vi "niRFUtil RFHS Channelizer ClearBuffer CSG.vi"(0 "Buffer":csg[](array[numeric]), 11 "error in (no error)":errorcluster) -> (15 "error out":errorcluster)   [LabVIEW 2015, in "niRFUtil.lvlib"]
uses:
  niRFUtil.lvlib
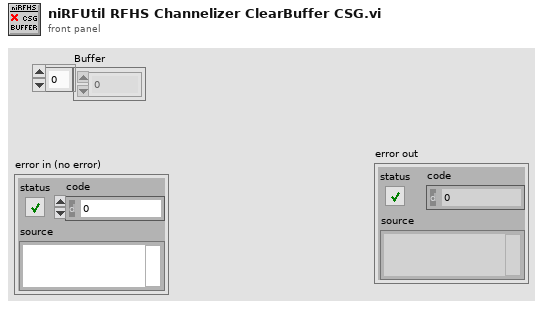
[diagram p1: front panel]
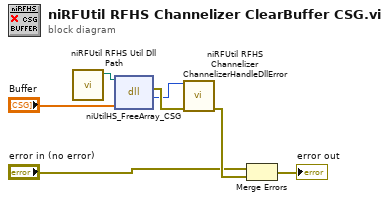
[diagram p0: block diagram]
diagram:
  n1 = call "niRFUtil RFHS Util Dll Path.vi"() -> ("Path"=w6:path)  [unwired: 7 in, 4 out]
  n2 = dll-call lib="?" fn="niUtilHS_FreeArray_CSG"(path in=w6, "buf"="Buffer") -> (error out=w5:errorcluster, "return type"=w4:i32)  [unwired: 3 in, 1 out]
  n3 = call "niRFUtil RFHS Channelizer ChannelizerHandleDllError.vi"("Error"=w4, "error in (no error)"=w5) -> ("error out"=w3:errorcluster)  [unwired: 13 in]
  n4 = Merge Errors("error in (no error)", w3) -> (→"error out":errorcluster)
